vi "Array Check.vi"(8 "Error In":errorcluster, 10 "Array Dimensions":i32[](array[numeric]), 11 "Vector Dimensions":T1={"Depth"=1, "Height"=1, "Width"=1} {"Width" min=1; "Height" min=1; "Depth" min=1}) -> (0 "error out":errorcluster, 3 "Smaller Array Size":u64)   [LabVIEW 2012, in "OpenCLV x64.lvlib"]
doc: "Checks if the vector dimensions are proper, see each case for details on what proper is."
uses:
  OpenCLV x64.lvlib
  User Controls/Array Dimensions.ctl
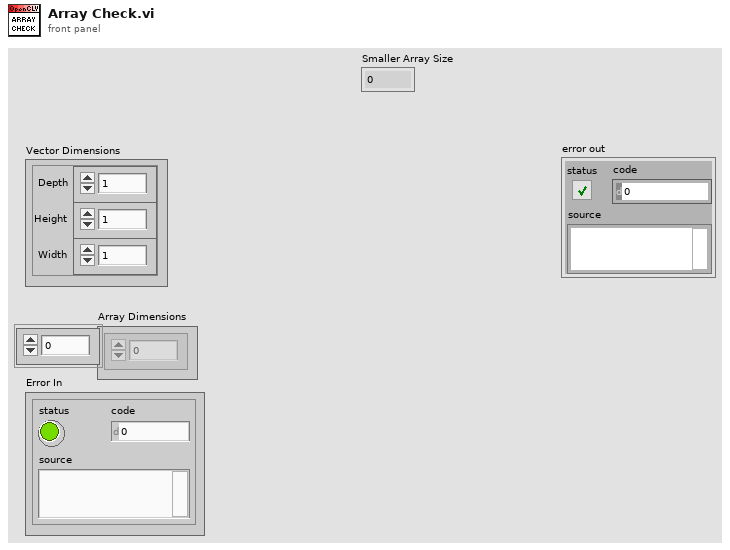
[diagram p1: front panel]
types:
  T1 = typedef "Array Dimensions.ctl" = cluster{"Depth":u64, "Height":u64, "Width":u64}
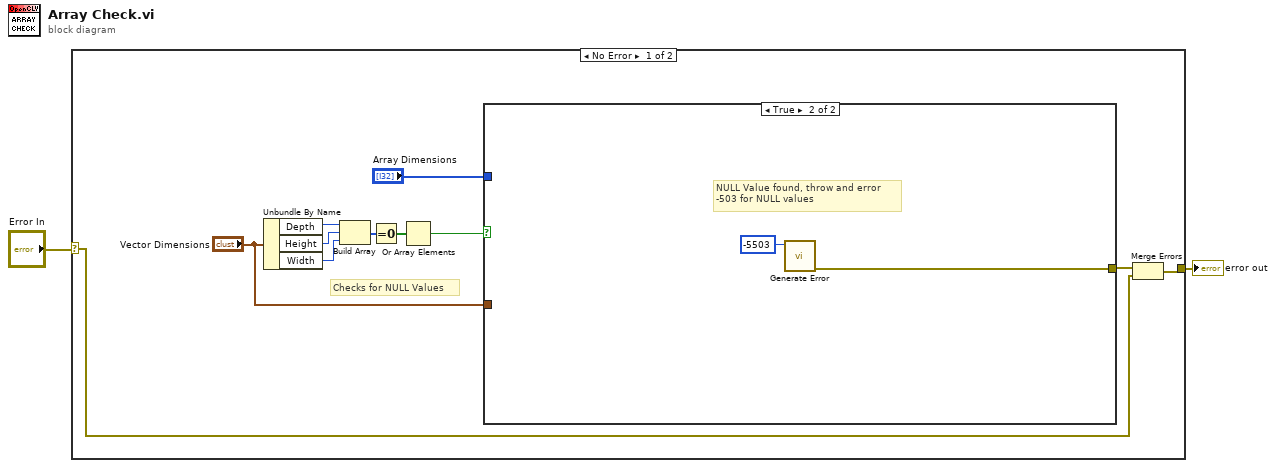
[diagram p0: block diagram]
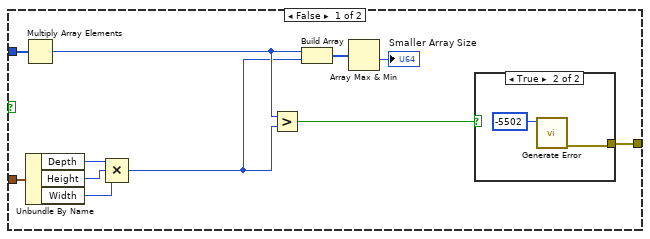
[diagram p2: hidden frame]
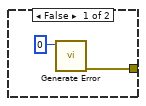
[diagram p3: hidden frame]
diagram:
  n1 = case shown="No Error" "Error In" {
    selector: "Error In" -> [w3 w31]
    tunnel: [w4 w31] -> w2
    frame No Error {
      # "Checks for NULL Values"
      n2 = Unbundle By Name("Vector Dimensions") -> ("Depth"=w11:u64, "Height"=w12:u64, "Width"=w13:u64)
      n3 = Build Array(w11, w12, w13) -> (w10:u64[])
      n4 = Equal To 0?(x=w10) -> (x = 0?=w9:bool[])
      n5 = Or Array Elements(Boolean array=w9) -> (logical OR=w8:bool)
      n6 = case shown="True" w8 {
        tunnel: [w24 w30] -> w5
        tunnel: "Vector Dimensions" -> [w23 _]
        tunnel: "Array Dimensions" -> [w19 _]
        frame False {
          n7 = Multiply Array Elements(1:w19) -> (0:w17:i32)
          n8 = Unbundle By Name(w23) -> ("Depth"=w22:u64, "Height"=w21:u64, "Width"=w20:u64)
          n9 = Compound Arithmetic op=MULTIPLY(w22, w21, w20) -> (w16:u64)
          n10 = Greater?(x=w17, y=w16) -> (0:w18:bool)
          n11 = Build Array(w17, w16) -> (w15:u64[])
          n12 = Array Max & Min(array=w15) -> (min value=→"Smaller Array Size":u64)  [unwired: 3 out]
          n13 = case shown="True" w18 {
            tunnel: [w25 w27] -> w24
            frame False {
              n14 = call "Generate Error.vi"("Error"=0) -> ("error out"=w25:errorcluster)  [unwired: 10 in]
            }
            frame True {
              n15 = call "Generate Error.vi"("Error"=-5502) -> ("error out"=w27:errorcluster)  [unwired: 10 in]
            }
          }
        }
        frame True {
          # "NULL Value found, throw and error\n-503 for NULL values"
          n16 = call "Generate Error.vi"("Error"=-5503) -> ("error out"=w30:errorcluster)  [unwired: 10 in]
        }
      }
      n17 = Merge Errors(w5, w3) -> (w4:errorcluster)
    }
    frame Error {
    }
  }
  "error out" <- w2
